vi "JSONtext Multi-step Filter.vi"() -> ()   [LabVIEW 2017] (continued)
53bcb93de39cd0c0af940\",\n    \"index\": 27,\n    \"guid\": \"0f0552d9-e7b3-4c57-b6c7-1e2135a1104f\",\n    \"isActive\": false,\n    \"balance\": \"$3,811.17\",\n    \"picture\": \"http://placehold.it/32x32\",\n    \"age\": 38,\n    \"eyeColor\": \"brown\",\n    \"name\": \"Merrill Ray\",\n    \"gender\": \"male\",\n    \"company\": \"SOLAREN\",\n    \"email\": \"merrillray@solaren.com\",\n    \"phone\": \"+1 (835) 524-2354\",\n    \"address\": \"227 Seacoast Terrace, Waterford, Kansas, 9740\",\n    \"about\": \"Magna eiusmod duis pariatur eiusmod minim et officia sit amet ipsum ut sint magna Lorem. Nisi velit sit adipisicing deserunt voluptate consectetur dolor officia voluptate elit adipisicing sit. Sint dolore occaecat ea duis voluptate duis sint ullamco in quis pariatur irure. Ipsum magna voluptate nulla deserunt eiusmod consectetur ut tempor qui pariatur quis duis. Lorem dolore qui adipisicing pariatur mollit cillum sunt nisi id deserunt tempor nisi amet. Sit cillum nisi dolore magna exercitation anim ad id consequat duis.\\r\\n\",\n    \"registered\": \"2016-06-15T02:30:18 -01:00\",\n    \"latitude\": 82.245484,\n    \"longitude\": -22.28782,\n    \"tags\": [\n      \"quis\",\n      \"pariatur\",\n      \"nisi\",\n      \"culpa\",\n      \"ut\",\n      \"minim\",\n      \"amet\"\n    ],\n    \"friends\": [\n      {\n        \"id\": 0,\n        \"name\": \"Fleming Rosario\"\n      },\n      {\n        \"id\": 1,\n        \"name\": \"Mcconnell Griffin\"\n      },\n      {\n        \"id\": 2,\n        \"name\": \"Marian Bradley\"\n      }\n    ],\n    \"greeting\": \"Hello, Merrill Ray! You have 3 unread messages.\",\n    \"favoriteFruit\": \"strawberry\"\n  },\n  {\n    \"_id\": \"59b53bcb56ebb2118edadabb\",\n    \"index\": 28,\n    \"guid\": \"31fd77e0-df37-4030-b598-6469f87deaaa\",\n    \"isActive\": false,\n    \"balance\": \"$1,128.38\",\n    \"picture\": \"http://placehold.it/32x32\",\n    \"age\": 22,\n    \"eyeColor\": \"green\",\n    \"name\": \"Cunningham Blevins\",\n    \"gender\": \"male\",\n    \"company\": \"SHOPABOUT\",\n    \"email\": \"cunninghamblevins@shopabout.com\",\n    \"phone\": \"+1 (960) 458-2822\",\n    \"address\": \"730 Llama Court, Riner, Puerto Rico, 7836\",\n    \"about\": \"Dolor quis officia nulla dolor amet sint excepteur enim esse est do. Eu ex ut aliquip velit do sint ullamco laborum. Occaecat eiusmod eiusmod velit adipisicing sit. Mollit eu pariatur eu consequat dolore irure fugiat sunt eiusmod cillum duis adipisicing eiusmod. Do commodo nisi irure cillum magna nulla enim aliqua dolor ullamco dolore pariatur.\\r\\n\",\n    \"registered\": \"2016-09-06T04:22:46 -01:00\",\n    \"latitude\": 83.759644,\n    \"longitude\": -43.131498,\n    \"tags\": [\n      \"velit\",\n      \"fugiat\",\n      \"dolor\",\n      \"ad\",\n      \"elit\",\n      \"dolore\",\n      \"ea\"\n    ],\n    \"friends\": [\n      {\n        \"id\": 0,\n        \"name\": \"Sanford Shannon\"\n      },\n      {\n        \"id\": 1,\n        \"name\": \"Burt Cherry\"\n      },\n      {\n        \"id\": 2,\n        \"name\": \"Kline Hale\"\n      }\n    ],\n    \"greeting\": \"Hello, Cunningham Blevins! You have 10 unread messages.\",\n    \"favoriteFruit\": \"strawberry\"\n  },\n  {\n    \"_id\": \"59b53bcb90a0cd7d08d9bf70\",\n    \"index\": 29,\n    \"guid\": \"8fb07447-f204-4b08-975d-44052bc193eb\",\n    \"isActive\": false,\n    \"balance\": \"$3,739.37\",\n    \"picture\": \"http://placehold.it/32x32\",\n    \"age\": 36,\n    \"eyeColor\": \"brown\",\n    \"name\": \"Bonner Lane\",\n    \"gender\": \"male\",\n    \"company\": \"COMVEY\",\n    \"email\": \"bonnerlane@comvey.com\",\n    \"phone\": \"+1 (847) 514-2794\",\n    \"address\": \"269 Dupont Street, Cedarville, South Carolina, 6587\",\n    \"about\": \"Velit Lorem magna deserunt minim ea exercitation quis veniam. Culpa cillum do aliquip exercitation enim aute in incididunt nostrud esse nostrud ullamco in. Amet mollit laborum eu laborum magna. Duis ad proident cillum esse fugiat enim est sit commodo. Dolore consectetur ut duis deserunt elit aliqua ad fugiat consectetur. Est aute aliquip ea consequat reprehenderit eiusmod. Consectetur tempor consequat duis voluptate mollit elit labore voluptate do cillum ex.\\r\\n\",\n    \"registered\": \"2017-02-20T02:31:32 -00:00\",\n    \"latitude\": -71.168208,\n    \"longitude\": -127.709761,\n    \"tags\": [\n      \"voluptate\",\n      \"consequat\",\n      \"incididunt\",\n      \"occaecat\",\n      \"amet\",\n      \"consequat\",\n      \"id\"\n    ],\n    \"friends\": [\n      {\n        \"id\": 0,\n        \"name\": \"Josie Horne\"\n      },\n      {\n        \"id\": 1,\n        \"name\": \"Nichole Weiss\"\n      },\n      {\n        \"id\": 2,\n        \"name\": \"Kristina Davidson\"\n      }\n    ],\n    \"greeting\": \"Hello, Bonner Lane! You have 3 unread messages.\",\n    \"favoriteFruit\": \"apple\"\n  },\n  {\n    \"_id\": \"59b53bcb35a25f2270b16071\",\n    \"index\": 30,\n    \"guid\": \"267938cb-8119-471f-85af-aa7a668d65fd\",\n    \"isActive\": false,\n    \"balance\": \"$2,354.36\",\n    \"picture\": \"http://placehold.it/32x32\",\n    \"age\": 35,\n    \"eyeColor\": \"blue\",\n    \"name\": \"Nielsen Burnett\",\n    \"gender\": \"male\",\n    \"company\": \"TURNABOUT\",\n    \"email\": \"nielsenburnett@turnabout.com\",\n    \"phone\": \"+1 (901) 404-2369\",\n    \"address\": \"499 Hart Place, Chesterfield, Mississippi, 6896\",\n    \"about\": \"Sunt magna sint ea deserunt reprehenderit aliqua in et proident. Minim consectetur dolore et commodo. Voluptate consectetur qui occaecat dolore eiusmod proident fugiat aute nulla id ad culpa exercitation occaecat.\\r\\n\",\n    \"registered\": \"2015-02-20T12:03:11 -00:00\",\n    \"latitude\": -46.775808,\n    \"longitude\": 173.193033,\n    \"tags\": [\n      \"enim\",\n      \"dolor\",\n      \"duis\",\n      \"Lorem\",\n      \"in\",\n      \"reprehenderit\",\n      \"ullamco\"\n    ],\n    \"friends\": [\n      {\n        \"id\": 0,\n        \"name\": \"Barlow Mcfadden\"\n      },\n      {\n        \"id\": 1,\n        \"name\": \"Clarissa Charles\"\n      },\n      {\n        \"id\": 2,\n        \"name\": \"Bray Patel\"\n      }\n    ],\n    \"greeting\": \"Hello, Nielsen Burnett! You have 7 unread messages.\",\n    \"favoriteFruit\": \"strawberry\"\n  },\n  {\n    \"_id\": \"59b53bcbe85d478fcadd3603\",\n    \"index\": 31,\n    \"guid\": \"3be04d8f-e807-4ad6-8ebd-c23cdbfe3dc4\",\n    \"isActive\": false,\n    \"balance\": \"$1,972.40\",\n    \"picture\": \"http://placehold.it/32x32\",\n    \"age\": 37,\n    \"eyeColor\": \"blue\",\n    \"name\": \"Elaine Allison\",\n    \"gender\": \"female\",\n    \"company\": \"QUANTASIS\",\n    \"email\": \"elaineallison@quantasis.com\",\n    \"phone\": \"+1 (981) 596-2824\",\n    \"address\": \"921 Kent Avenue, Breinigsville, Wisconsin, 3750\",\n    \"about\": \"Minim cillum ea irure officia. Irure in dolor ea veniam adipisicing sint nisi amet ipsum excepteur nisi excepteur est deserunt. Consequat voluptate mollit sint magna Lorem in nulla proident Lorem. Proident est id esse ad ea. Dolore Lorem aliquip officia veniam anim velit et id ullamco et dolor eu aliqua quis. Dolore magna est mollit in ut ea voluptate nostrud do aliquip. In reprehenderit non eiusmod veniam ex.\\r\\n\",\n    \"registered\": \"2017-03-24T04:15:39 -00:00\",\n    \"latitude\": 7.656665,\n    \"longitude\": 56.755826,\n    \"tags\": [\n      \"nisi\",\n      \"labore\",\n      \"fugiat\",\n      \"ex\",\n      \"reprehenderit\",\n      \"nisi\",\n      \"sint\"\n    ],\n    \"friends\": [\n      {\n        \"id\": 0,\n        \"name\": \"Alta Bruce\"\n      },\n      {\n        \"id\": 1,\n        \"name\": \"Cora Ruiz\"\n      },\n      {\n        \"id\": 2,\n        \"name\": \"Mercer Barron\"\n      }\n    ],\n    \"greeting\": \"Hello, Elaine Allison! You have 1 unread messages.\",\n    \"favoriteFruit\": \"banana\"\n  },\n  {\n    \"_id\": \"59b53bcbf5dcc9341b3c298d\",\n    \"index\": 32,\n    \"guid\": \"bf62375b-123f-4c02-85e3-3a78c18e6f70\",\n    \"isActive\": false,\n    \"balance\": \"$1,895.96\",\n    \"picture\": \"http://placehold.it/32x32\",\n    \"age\": 28,\n    \"eyeColor\": \"brown\",\n    \"name\": \"Christa Robertson\",\n    \"gender\": \"female\",\n    \"company\": \"ICOLOGY\",\n    \"email\": \"christarobertson@icology.com\",\n    \"phone\": \"+1 (888) 410-3337\",\n    \"address\": \"989 Clara Street, Ogema, Indiana, 2922\",\n    \"about\": \"Enim mollit officia occaecat non nostrud ad cupidatat amet. Sunt ipsum proident consectetur voluptate id excepteur id magna. Do commodo culpa id esse officia cupidatat dolore duis non laboris veniam. Laboris ad dolor qui anim et ut dolor excepteur irure elit adipisicing ex labore eiusmod. Sunt minim velit nostrud irure quis consequat officia fugiat amet ipsum. Nostrud laboris do fugiat proident reprehenderit duis exercitation aute enim ex ullamco proident. Qui sint adipisicing occaecat aliqua non culpa esse id dolor voluptate ipsum deserunt in.\\r\\n\",\n    \"registered\": \"2015-02-16T07:12:55 -00:00\",\n    \"latitude\": 52.102423,\n    \"longitude\": -24.794434,\n    \"tags\": [\n      \"dolore\",\n      \"fugiat\",\n      \"aliqua\",\n      \"minim\",\n      \"pariatur\",\n      \"laborum\",\n      \"qui\"\n    ],\n    \"friends\": [\n      {\n        \"id\": 0,\n        \"name\": \"Cathy Cohen\"\n      },\n      {\n        \"id\": 1,\n        \"name\": \"Shawna Green\"\n      },\n      {\n        \"id\": 2,\n        \"name\": \"Ward Mckay\"\n      }\n    ],\n    \"greeting\": \"Hello, Christa Robertson! You have 9 unread messages.\",\n    \"favoriteFruit\": \"banana\"\n  },\n  {\n    \"_id\": \"59b53bcb8f369a2e50811288\",\n    \"index\": 33,\n    \"guid\": \"74275f14-281e-4519-a0c4-b708fa901d88\",\n    \"isActive\": true,\n    \"balance\": \"$2,269.82\",\n    \"picture\": \"http://placehold.it/32x32\",\n    \"age\": 36,\n    \"eyeColor\": \"green\",\n    \"name\": \"Castillo Kerr\",\n    \"gender\": \"male\",\n    \"company\": \"ZENTHALL\",\n    \"email\": \"castillokerr@zenthall.com\",\n    \"phone\": \"+1 (964) 406-2670\",\n    \"address\": \"210 Campus Road, Templeton, Tennessee, 2482\",\n    \"about\": \"Irure ut nisi adipisicing non duis mollit. Tempor deserunt ut nostrud ipsum enim dolore Lorem labore. Duis sint magna nisi et anim ex. Ea eu exercitation est laboris nostrud qui eiusmod. Ullamco amet ut Lorem eu adipisicing incididunt qui aliquip pariatur sint proident anim voluptate veniam. Excepteur aute velit deserunt deserunt et ex elit excepteur enim reprehenderit. Commodo ad aliquip Lorem excepteur reprehenderit quis in ea sint esse proident.\\r\\n\",\n    \"registered\": \"2016-05-03T04:24:26 -01:00\",\n    \"latitude\": -38.877683,\n    \"longitude\": -171.766918,\n    \"tags\": [\n      \"officia\",\n      \"aliquip\",\n      \"consequat\",\n      \"voluptate\",\n      \"cillum\",\n      \"do\",\n      \"officia\"\n    ],\n    \"friends\": [\n      {\n        \"id\": 0,\n        \"name\": \"Cara Hoffman\"\n      },\n      {\n        \"id\": 1,\n        \"name\": \"Joyner Beasley\"\n      },\n      {\n        \"id\": 2,\n        \"name\": \"Lucy Grimes\"\n      }\n    ],\n    \"greeting\": \"Hello, Castillo Kerr! You have 9 unread messages.\",\n    \"favoriteFruit\": \"strawberry\"\n  },\n  {\n    \"_id\": \"59b53bcbb2ac6162cf8d89a7\",\n    \"index\": 34,\n    \"guid\": \"3d62cd17-ac67-4b71-a5da-4ccef6cce1d0\",\n    \"isActive\": false,\n    \"balance\": \"$1,731.00\",\n    \"picture\": \"http://placehold.it/32x32\",\n    \"age\": 24,\n    \"eyeColor\": \"blue\",\n    \"name\": \"Melissa Gregory\",\n    \"gender\": \"female\",\n    \"company\": \"UPLINX\",\n    \"email\": \"melissagregory@uplinx.com\",\n    \"phone\": \"+1 (907) 532-2994\",\n    \"address\": \"394 Miller Avenue, Cashtown, Georgia, 520\",\n    \"about\": \"Consequat mollit occaecat proident officia reprehenderit. Ipsum minim ex reprehenderit et reprehenderit sunt. Esse ea quis nulla do. Cupidatat sit et tempor tempor voluptate qui est ad. Ad magna adipisicing excepteur excepteur ad quis. Fugiat laborum adipisicing do commodo ex qui ut minim ipsum commodo irure ex ea. Fugiat ad anim dolor do adipisicing veniam laboris laboris nostrud reprehenderit mollit eiusmod dolore laboris.\\r\\n\",\n    \"registered\": \"2016-03-22T12:23:21 -00:00\",\n    \"latitude\": -13.24058,\n    \"longitude\": 174.343852,\n    \"tags\": [\n      \"aliqua\",\n      \"veniam\",\n      \"do\",\n      \"tempor\",\n      \"voluptate\",\n      \"officia\",\n      \"id\"\n    ],\n    \"friends\": [\n      {\n        \"id\": 0,\n        \"name\": \"Mccall Baker\"\n      },\n      {\n        \"id\": 1,\n        \"name\": \"Elena Raymond\"\n      },\n      {\n        \"id\": 2,\n        \"name\": \"Harvey Hubbard\"\n      }\n    ],\n    \"greeting\": \"Hello, Melissa Gregory! You have 7 unread messages.\",\n    \"favoriteFruit\": \"banana\"\n  },\n  {\n    \"_id\": \"59b53bcb9bea1476ae4824c8\",\n    \"index\": 35,\n    \"guid\": \"705c7090-a759-43dc-b18c-63ad736d29ca\",\n    \"isActive\": false,\n    \"balance\": \"$2,004.78\",\n    \"picture\": \"http://placehold.it/32x32\",\n    \"age\": 37,\n    \"eyeColor\": \"brown\",\n    \"name\": \"Lancaster Welch\",\n    \"gender\": \"male\",\n    \"company\": \"JIMBIES\",\n    \"email\": \"lancasterwelch@jimbies.com\",\n    \"phone\": \"+1 (961) 509-2893\",\n    \"address\": \"477 Crystal Street, Lindcove, New Hampshire, 655\",\n    \"about\": \"Anim ex duis laboris non ullamco non deserunt magna ex voluptate mollit in excepteur. Sit excepteur proident ad magna esse elit veniam qui ad veniam cupidatat non duis. Eiusmod laboris id cupidatat exercitation quis adipisicing sunt eiusmod enim magna. Qui aliqua qui dolore enim veniam consequat ea cillum cupidatat voluptate excepteur in. Eu culpa anim veniam nisi officia consectetur ut exercitation fugiat quis sit ipsum enim quis. Lorem ut magna in sit.\\r\\n\",\n    \"registered\": \"2016-07-01T05:06:00 -01:00\",\n    \"latitude\": 29.49636,\n    \"longitude\": -45.617538,\n    \"tags\": [\n      \"adipisicing\",\n      \"enim\",\n      \"do\",\n      \"culpa\",\n      \"esse\",\n      \"proident\",\n      \"velit\"\n    ],\n    \"friends\": [\n      {\n        \"id\": 0,\n        \"name\": \"Whitehead Moss\"\n      },\n      {\n        \"id\": 1,\n        \"name\": \"Melisa Bridges\"\n      },\n      {\n        \"id\": 2,\n        \"name\": \"Helene Barrett\"\n      }\n    ],\n    \"greeting\": \"Hello, Lancaster Welch! You have 4 unread messages.\",\n    \"favoriteFruit\": \"strawberry\"\n  },\n  {\n    \"_id\": \"59b53bcb1dfb6733db2fc827\",\n    \"index\": 36,\n    \"guid\": \"0d80f8b7-650a-4492-b9ae-8c5d36bf2d83\",\n    \"isActive\": true,\n    \"balance\": \"$3,087.53\",\n    \"picture\": \"http://placehold.it/32x32\",\n    \"age\": 21,\n    \"eyeColor\": \"brown\",\n    \"name\": \"Clemons Juarez\",\n    \"gender\": \"male\",\n    \"company\": \"EMERGENT\",\n    \"email\": \"clemonsjuarez@emergent.com\",\n    \"phone\": \"+1 (899) 574-2444\",\n    \"address\": \"962 Seagate Avenue, Diaperville, Louisiana, 9282\",\n    \"about\": \"Labore adipisicing in enim eu laboris veniam minim sit do velit. Nulla amet ullamco anim cupidatat. Aliquip officia laborum nulla nisi aliqua dolore elit aute tempor ut culpa commodo. Esse cupidatat officia pariatur pariatur.\\r\\n\",\n    \"registered\": \"2015-07-29T04:09:12 -01:00\",\n    \"latitude\": 16.025236,\n    \"longitude\": -68.678922,\n    \"tags\": [\n      \"et\",\n      \"sunt\",\n      \"enim\",\n      \"dolor\",\n      \"labore\",\n      \"nostrud\",\n      \"adipisicing\"\n    ],\n    \"friends\": [\n      {\n        \"id\": 0,\n        \"name\": \"Dorothea Barnett\"\n      },\n      {\n        \"id\": 1,\n        \"name\": \"Terrie Knox\"\n      },\n      {\n        \"id\": 2,\n        \"name\": \"Dodson Dale\"\n      }\n    ],\n    \"greeting\": \"Hello, Clemons Juarez! You have 7 unread messages.\",\n    \"favoriteFruit\": \"apple\"\n  },\n  {\n    \"_id\": \"59b53bcba7232f419ad64f14\",\n    \"index\": 37,\n    \"guid\": \"15bec63f-2a77-45db-a3cf-11092f20cb9e\",\n    \"isActive\": false,\n    \"balance\": \"$3,716.74\",\n    \"picture\": \"http://placehold.it/32x32\",\n    \"age\": 29,\n    \"eyeColor\": \"green\",\n    \"name\": \"Hillary Waller\",\n    \"gender\": \"female\",\n    \"company\": \"MUSIX\",\n    \"email\": \"hillarywaller@musix.com\",\n    \"phone\": \"+1 (947) 549-3976\",\n    \"address\": \"601 Kay Court, Rockhill, Oklahoma, 5198\",\n    \"about\": \"Sit reprehenderit ad mollit reprehenderit do aliquip fugiat aute consectetur eu excepteur eiusmod dolor Lorem. Deserunt consectetur ex et deserunt velit quis excepteur labore deserunt cillum. Dolore mollit qui proident minim eiusmod.\\r\\n\",\n    \"registered\": \"2015-10-22T03:23:57 -01:00\",\n    \"latitude\": 2.128634,\n    \"longitude\": 43.198503,\n    \"tags\": [\n      \"duis\",\n      \"non\",\n      \"dolore\",\n      \"aliqua\",\n      \"culpa\",\n      \"proident\",\n      \"sint\"\n    ],\n    \"friends\": [\n      {\n        \"id\": 0,\n        \"name\": \"Vega Lawson\"\n      },\n      {\n        \"id\": 1,\n        \"name\": \"Phelps Wolf\"\n      },\n      {\n        \"id\": 2,\n        \"name\": \"Gloria Mcmillan\"\n      }\n    ],\n    \"greeting\": \"Hello, Hillary Waller! You have 10 unread messages.\",\n    \"favoriteFruit\": \"apple\"\n  },\n  {\n    \"_id\": \"59b53bcb1344ea6331b52625\",\n    \"index\": 38,\n    \"guid\": \"561edd27-6d57-4a6f-956c-f3bf54efe435\",\n    \"isActive\": true,\n    \"balance\": \"$3,213.23\",\n    \"picture\": \"http://placehold.it/32x32\",\n    \"age\": 32,\n    \"eyeColor\": \"brown\",\n    \"name\": \"Jackie Lott\",\n    \"gender\": \"female\",\n    \"company\": \"ORBIN\",\n    \"email\": \"jackielott@orbin.com\",\n    \"phone\": \"+1 (825) 509-2344\",\n    \"address\": \"921 Frost Street, Dubois, Alaska, 1796\",\n    \"about\": \"Reprehenderit veniam Lorem ea do proident in fugiat aliqua. Id proident nostrud aliqua tempor reprehenderit eiusmod ullamco velit duis. Anim ipsum nulla reprehenderit do exercitation consequat nisi in commodo qui fugiat nostrud.\\r\\n\",\n    \"registered\": \"2017-08-19T04:32:54 -01:00\",\n    \"latitude\": 23.292166,\n    \"longitude\": 35.845555,\n    \"tags\": [\n      \"dolore\",\n      \"veniam\",\n      \"labore\",\n      \"et\",\n      \"culpa\",\n      \"est\",\n      \"officia\"\n    ],\n    \"friends\": [\n      {\n        \"id\": 0,\n        \"name\": \"Diaz Warren\"\n      },\n      {\n        \"id\": 1,\n        \"name\": \"Sullivan Watkins\"\n      },\n      {\n        \"id\": 2,\n        \"name\": \"Maynard Page\"\n      }\n    ],\n    \"greeting\": \"Hello, Jackie Lott! You have 4 unread messages.\",\n    \"favoriteFruit\": \"apple\"\n  },\n  {\n    \"_id\": \"59b53bcb21e1aba2d54ad2f8\",\n    \"index\": 39,\n    \"guid\": \"c9ee8206-d3bd-48ae-9fda-5b5529ac4057\",\n    \"isActive\": false,\n    \"balance\": \"$3,035.61\",\n    \"picture\": \"http://placehold.it/32x32\",\n    \"age\": 29,\n    \"eyeColor\": \"green\",\n    \"name\": \"Flynn Pruitt\",\n    \"gender\": \"male\",\n    \"company\": \"ORBEAN\",\n    \"email\": \"flynnpruitt@orbean.com\",\n    \"phone\": \"+1 (866) 596-2533\",\n    \"address\": \"274 Ridgewood Place, Durham, North Dakota, 3534\",\n    \"about\": \"Commodo sint irure deserunt Lorem laboris laborum mollit ea ipsum incididunt laboris adipisicing proident. Velit tempor minim et occaecat exercitation et commodo consequat velit. Minim irure esse ullamco commodo labore ex mollit esse. Ipsum nostrud est ex Lorem culpa.\\r\\n\",\n    \"registered\": \"2015-06-20T09:17:37 -01:00\",\n    \"latitude\": -50.018521,\n    \"longitude\": 165.121492,\n    \"tags\": [\n      \"irure\",\n      \"ea\",\n      \"quis\",\n      \"dolore\",\n      \"irure\",\n      \"aliqua\",\n      \"pariatur\"\n    ],\n    \"friends\": [\n      {\n        \"id\": 0,\n        \"name\": \"Carla Snow\"\n      },\n      {\n        \"id\": 1,\n        \"name\": \"Cochran Thomas\"\n      },\n      {\n        \"id\": 2,\n        \"name\": \"Guy Roberts\"\n      }\n    ],\n    \"greeting\": \"Hello, Flynn Pruitt! You have 10 unread messages.\",\n    \"favoriteFruit\": \"banana\"\n  },\n  {\n    \"_id\": \"59b53bcb88a5fd7e5b5805c7\",\n    \"index\": 40,\n    \"guid\": \"ef10c0b3-7ab0-4313-b2b2-462164f5485a\",\n    \"isActive\": true,\n    \"balance\": \"$1,173.28\",\n    \"picture\": \"http://placehold.it/32x32\",\n    \"age\": 39,\n    \"eyeColor\": \"brown\",\n    \"name\": \"Shelby Albert\",\n    \"gender\": \"female\",\n    \"company\": \"HYDROCOM\",\n    \"email\": \"shelbyalbert@hydrocom.com\",\n    \"phone\": \"+1 (977) 400-2351\",\n    \"address\": \"393 Glendale Court, Catharine, Washington, 6629\",\n    \"about\": \"Do laborum exercitation eiusmod sunt esse laboris qui Lorem dolor amet consectetur id. Officia est exercitation proident pariatur culpa ea sint veniam reprehenderit aliquip. Laborum dolore ad mollit nostrud cillum ad tempor anim occaecat sit. Amet consequat eiusmod laboris consectetur.\\r\\n\",\n    \"registered\": \"2015-07-17T06:49:02 -01:00\",\n    \"latitude\": -32.156776,\n    \"longitude\": -68.42255,\n    \"tags\": [\n      \"laborum\",\n      \"dolor\",\n      \"sit\",\n      \"sit\",\n      \"ad\",\n      \"sunt\",\n      \"minim\"\n    ],\n    \"friends\": [\n      {\n        \"id\": 0,\n        \"name\": \"Huber Hahn\"\n      },\n      {\n        \"id\": 1,\n        \"name\": \"Felicia Mooney\"\n      },\n      {\n        \"id\": 2,\n        \"name\": \"Kathryn Alvarado\"\n      }\n    ],\n    \"greeting\": \"Hello, Shelby Albert! You have 1 unread messages.\",\n    \"favoriteFruit\": \"banana\"\n  },\n  {\n    \"_id\": \"59b53bcbacd63a0258d513a3\",\n    \"index\": 41,\n    \"guid\": \"7142ec6a-9741-41fd-8c8f-fba9cc5ff0ab\",\n    \"isActive\": true,\n    \"balance\": \"$3,196.96\",\n    \"picture\": \"http://placehold.it/32x32\",\n    \"age\": 34,\n    \"eyeColor\": \"brown\",\n    \"name\": \"Bailey Snyder\",\n    \"gender\": \"male\",\n    \"company\": \"ISOSURE\",\n    \"email\": \"baileysnyder@isosure.com\",\n    \"phone\": \"+1 (976) 469-3334\",\n    \"address\": \"754 Emerson Place, Stagecoach, New York, 1029\",\n    \"about\": \"Veniam dolore qui elit ea qui ipsum exercitation sunt sunt in ad mollit. Excepteur adipisicing et consectetur proident veniam laborum adipisicing consectetur eiusmod. Culpa consequat officia ipsum nisi proident proident velit. Fugiat commodo ad do commodo tempor proident excepteur mollit magna.\\r\\n\",\n    \"registered\": \"2015-09-25T01:25:56 -01:00\",\n    \"latitude\": -76.0324,\n    \"longitude\": -73.748444,\n    \"tags\": [\n      \"minim\",\n      \"adipisicing\",\n      \"Lorem\",\n      \"eu\",\n      \"ex\",\n      \"deserunt\",\n      \"eu\"\n    ],\n    \"friends\": [\n      {\n        \"id\": 0,\n        \"name\": \"Waters Hartman\"\n      },\n      {\n        \"id\": 1,\n        \"name\": \"Valdez Baird\"\n      },\n      {\n        \"id\": 2,\n        \"name\": \"Serena Mills\"\n      }\n    ],\n    \"greeting\": \"Hello, Bailey Snyder! You have 5 unread messages.\",\n    \"favoriteFruit\": \"strawberry\"\n  },\n  {\n    \"_id\": \"59b53bcba4a6b906f6c552ad\",\n    \"index\": 42,\n    \"guid\": \"46d7ec6e-a1f2-4133-bd5d-cc56e5102a00\",\n    \"isActive\": true,\n    \"balance\": \"$3,341.48\",\n    \"picture\": \"http://placehold.it/32x32\",\n    \"age\": 32,\n    \"eyeColor\": \"brown\",\n    \"name\": \"Erika Porter\",\n    \"gender\": \"female\",\n    \"company\": \"ZENTIME\",\n    \"email\": \"erikaporter@zentime.com\",\n    \"phone\": \"+1 (937) 468-3114\",\n    \"address\": \"917 Ovington Avenue, Stouchsburg, Alabama, 9680\",\n    \"about\": \"Consectetur reprehenderit nisi cupidatat deserunt nulla laboris ut. Nisi deserunt dolore occaecat fugiat esse pariatur quis non commodo laboris elit voluptate. Nulla ex laborum Lorem ipsum incididunt reprehenderit elit dolore ullamco amet duis esse est ullamco. Enim in mollit labore laborum sunt.\\r\\n\",\n    \"registered\": \"2015-01-22T11:40:33 -00:00\",\n    \"latitude\": 53.845955,\n    \"longitude\": -126.430992,\n    \"tags\": [\n      \"incididunt\",\n      \"elit\",\n      \"duis\",\n      \"deserunt\",\n      \"sint\",\n      \"labore\",\n      \"irure\"\n    ],\n    \"friends\": [\n      {\n        \"id\": 0,\n        \"name\": \"Monica Lyons\"\n      },\n      {\n        \"id\": 1,\n        \"name\": \"Katrina Brennan\"\n      },\n      {\n        \"id\": 2,\n        \"name\": \"Kim Francis\"\n      }\n    ],\n    \"greeting\": \"Hello, Erika Porter! You have 4 unread messages.\",\n    \"favoriteFruit\": \"strawberry\"\n  },\n  {\n    \"_id\": \"59b53bcb1c73edcfc9efe849\",\n    \"index\": 43,\n    \"guid\": \"84a42cb7-4fea-42c7-961d-2535547c818b\",\n    \"isActive\": true,\n    \"balance\": \"$1,840.08\",\n    \"picture\": \"http://placehold.it/32x32\",\n    \"age\": 29,\n    \"eyeColor\": \"brown\",\n    \"name\": \"Marjorie Craig\",\n    \"gender\": \"female\",\n    \"company\": \"PROGENEX\",\n    \"email\": \"marjoriecraig@progenex.com\",\n    \"phone\": \"+1 (898) 534-3929\",\n    \"address\": \"262 Exeter Street, Elliott, Arkansas, 9839\",\n    \"about\": \"Ipsum esse irure dolor consectetur amet ullamco. Ut nostrud anim occaecat dolor dolor sit adipisicing cupidatat. Veniam velit pariatur id magna in sit.\\r\\n\",\n    \"registered\": \"2014-11-10T05:13:50 -00:00\",\n    \"latitude\": 74.482858,\n    \"longitude\": 69.078973,\n    \"tags\": [\n      \"excepteur\",\n      \"cillum\",\n      \"minim\",\n      \"aliqua\",\n      \"exercitation\",\n      \"incididunt\",\n      \"dolor\"\n    ],\n    \"friends\": [\n      {\n        \"id\": 0,\n        \"name\": \"Horton Taylor\"\n      },\n      {\n        \"id\": 1,\n        \"name\": \"Melinda Ashley\"\n      },\n      {\n        \"id\": 2,\n        \"name\": \"Margie Roy\"\n      }\n    ],\n    \"greeting\": \"Hello, Marjorie Craig! You have 6 unread messages.\",\n    \"favoriteFruit\": \"banana\"\n  },\n  {\n    \"_id\": \"59b53bcb2edcfd9a5f058115\",\n    \"index\": 44,\n    \"guid\": \"8101a8ef-a578-4a86-9b90-204b2b6ca3bc\",\n    \"isActive\": false,\n    \"balance\": \"$1,295.45\",\n    \"picture\": \"http://placehold.it/32x32\",\n    \"age\": 20,\n    \"eyeColor\": \"blue\",\n    \"name\": \"Tina Browning\",\n    \"gender\": \"female\",\n    \"company\": \"KNOWLYSIS\",\n    \"email\": \"tinabrowning@knowlysis.com\",\n    \"phone\": \"+1 (878) 557-2240\",\n    \"address\": \"470 Lawton Street, Avoca, Northern Mariana Islands, 1174\",\n    \"about\": \"Officia quis reprehenderit eiusmod sit mollit duis minim duis elit exercitation sunt quis aliquip est. Velit esse occaecat irure deserunt amet dolore voluptate deserunt exercitation id. Dolor culpa dolor adipisicing do irure. Ullamco incididunt elit non mollit excepteur nisi proident ut eu sit dolor excepteur. Reprehenderit Lorem adipisicing deserunt eu labore laborum cillum ullamco nisi esse magna. Amet et ad nisi ad elit velit in in sunt veniam occaecat pariatur quis exercitation.\\r\\n\",\n    \"registered\": \"2015-10-18T08:14:25 -01:00\",\n    \"latitude\": 35.369634,\n    \"longitude\": -88.568524,\n    \"tags\": [\n      \"eu\",\n      \"veniam\",\n      \"quis\",\n      \"sint\",\n      \"excepteur\",\n      \"fugiat\",\n      \"minim\"\n    ],\n    \"friends\": [\n      {\n        \"id\": 0,\n        \"name\": \"Yolanda Mcgee\"\n      },\n      {\n        \"id\": 1,\n        \"name\": \"Tara Rich\"\n      },\n      {\n        \"id\": 2,\n        \"name\": \"Walton Maynard\"\n      }\n    ],\n    \"greeting\": \"Hello, Tina Browning! You have 8 unread messages.\",\n    \"favoriteFruit\": \"apple\"\n  },\n  {\n    \"_id\": \"59b53bcb3e923247d8ec4740\",\n    \"index\": 45,\n    \"guid\": \"b966f77e-3e7a-4bc1-8268-d15e38d760e2\",\n    \"isActive\": false,\n    \"balance\": \"$1,071.05\",\n    \"picture\": \"http://placehold.it/32x32\",\n    \"age\": 34,\n    \"eyeColor\": \"blue\",\n    \"name\": \"Estela Morrison\",\n    \"gender\": \"female\",\n    \"company\": \"DELPHIDE\",\n    \"email\": \"estelamorrison@delphide.com\",\n    \"phone\": \"+1 (895) 541-2685\",\n    \"address\": \"492 Ryder Avenue, Sims, West Virginia, 7864\",\n    \"about\": \"Est aliqua sit consectetur do occaecat ullamco commodo fugiat et. Culpa amet ipsum enim quis duis exercitation non nisi adipisicing aliquip incididunt irure. Labore aliqua sint nulla reprehenderit in reprehenderit tempor ullamco quis ipsum. Fugiat irure ut sit adipisicing cillum magna ad sit enim elit irure. Proident aliqua eu et anim est reprehenderit fugiat non. Commodo enim id nulla sit nisi. Excepteur tempor officia ipsum in pariatur.\\r\\n\",\n    \"registered\": \"2015-01-29T12:06:00 -00:00\",\n    \"latitude\": -31.693065,\n    \"longitude\": -53.009874,\n    \"tags\": [\n      \"magna\",\n      \"consequat\",\n      \"enim\",\n      \"velit\",\n      \"anim\",\n      \"velit\",\n      \"ad\"\n    ],\n    \"friends\": [\n      {\n        \"id\": 0,\n        \"name\": \"Callahan King\"\n      },\n      {\n        \"id\": 1,\n        \"name\": \"Key Wallace\"\n      },\n      {\n        \"id\": 2,\n        \"name\": \"Carney Arnold\"\n      }\n    ],\n    \"greeting\": \"Hello, Estela Morrison! You have 3 unread messages.\",\n    \"favoriteFruit\": \"apple\"\n  },\n  {\n    \"_id\": \"59b53bcb1526a6fceba75760\",\n    \"index\": 46,\n    \"guid\": \"5ef8b250-99fd-4d8e-99c0-bb5f3d3bdac3\",\n    \"isActive\": false,\n    \"balance\": \"$2,675.97\",\n    \"picture\": \"http://placehold.it/32x32\",\n    \"age\": 31,\n    \"eyeColor\": \"green\",\n    \"name\": \"Adela Ryan\",\n    \"gender\": \"female\",\n    \"company\": \"FLUMBO\",\n    \"email\": \"adelaryan@flumbo.com\",\n    \"phone\": \"+1 (906) 429-3206\",\n    \"address\": \"952 Richmond Street, Rodanthe, South Dakota, 2236\",\n    \"about\": \"Ea non aliquip fugiat Lorem magna pariatur excepteur officia qui quis officia occaecat quis est. Amet incididunt nisi duis commodo sint cillum tempor. Minim reprehenderit ut Lorem labore eu magna proident voluptate occaecat amet quis. Ipsum nulla ullamco ad enim duis velit eiusmod consectetur aliqua ad. Nisi aliquip esse proident nostrud officia non sit laboris amet excepteur dolor commodo ad. Cillum velit et ad aliquip esse mollit in enim tempor dolor. Aliqua esse excepteur mollit mollit.\\r\\n\",\n    \"registered\": \"2014-08-15T04:54:20 -01:00\",\n    \"latitude\": 49.702844,\n    \"longitude\": 154.358542,\n    \"tags\": [\n      \"nostrud\",\n      \"non\",\n      \"laboris\",\n      \"nostrud\",\n      \"eu\",\n      \"adipisicing\",\n      \"ad\"\n    ],\n    \"friends\": [\n      {\n        \"id\": 0,\n        \"name\": \"Moss Bright\"\n      },\n      {\n        \"id\": 1,\n        \"name\": \"Houston Glass\"\n      },\n      {\n        \"id\": 2,\n        \"name\": \"Cherry Moon\"\n      }\n    ],\n    \"greeting\": \"Hello, Adela Ryan! You have 2 unread messages.\",\n    \"favoriteFruit\": \"apple\"\n  },\n  {\n    \"_id\": \"59b53bcbb6aeae8f27f300a9\",\n    \"index\": 47,\n    \"guid\": \"8e8ffd1c-34dd-4984-9245-b4713cc73b00\",\n    \"isActive\": true,\n    \"balance\": \"$3,353.90\",\n    \"picture\": \"http://placehold.it/32x32\",\n    \"age\": 36,\n    \"eyeColor\": \"blue\",\n    \"name\": \"Cote Barlow\",\n    \"gender\": \"male\",\n    \"company\": \"BEZAL\",\n    \"email\": \"cotebarlow@bezal.com\",\n    \"phone\": \"+1 (987) 473-2295\",\n    \"address\": \"560 Emmons Avenue, Wolcott, Delaware, 8148\",\n    \"about\": \"Qui aliqua sit laboris eu consectetur commodo qui ullamco cupidatat id enim ex sit. Anim reprehenderit tempor ut fugiat. Sunt et consequat proident proident. Irure sunt adipisicing commodo do enim exercitation fugiat aliqua consequat anim do et sint. Enim excepteur reprehenderit deserunt pariatur do voluptate ullamco aliqua magna labore deserunt tempor id. Enim dolor nostrud qui ullamco cillum officia mollit.\\r\\n\",\n    \"registered\": \"2014-04-10T08:27:55 -01:00\",\n    \"latitude\": 66.218671,\n    \"longitude\": 64.565323,\n    \"tags\": [\n      \"magna\",\n      \"reprehenderit\",\n      \"velit\",\n      \"nulla\",\n      \"aliqua\",\n      \"quis\",\n      \"nisi\"\n    ],\n    \"friends\": [\n      {\n        \"id\": 0,\n        \"name\": \"Stark Yates\"\n      },\n      {\n        \"id\": 1,\n        \"name\": \"Ginger Wilkinson\"\n      },\n      {\n        \"id\": 2,\n        \"name\": \"Bradford Durham\"\n      }\n    ],\n    \"greeting\": \"Hello, Cote Barlow! You have 10 unread messages.\",\n    \"favoriteFruit\": \"apple\"\n  },\n  {\n    \"_id\": \"59b53bcbb025a60e792d23e8\",\n    \"index\": 48,\n    \"guid\": \"399c42d0-8971-45d8-ac59-af2f1ffaebd0\",\n    \"isActive\": true,\n    \"balance\": \"$3,820.26\",\n    \"picture\": \"http://placehold.it/32x32\",\n    \"age\": 32,\n    \"eyeColor\": \"brown\",\n    \"name\": \"Higgins Randall\",\n    \"gender\": \"male\",\n    \"company\": \"ECSTASIA\",\n    \"email\": \"higginsrandall@ecstasia.com\",\n    \"phone\": \"+1 (895) 474-3692\",\n    \"address\": \"325 John Street, Welch, Nebraska, 2056\",\n    \"about\": \"Cupidatat non minim occaecat proident enim consectetur occaecat Lorem duis ut. Quis incididunt nostrud amet ut laborum consequat aliquip excepteur. Dolor ipsum aute consectetur id quis Lorem culpa nostrud sint ipsum esse reprehenderit aliqua. Dolor id ex consequat nisi quis esse officia veniam. Sit amet cillum ea irure consectetur exercitation laboris culpa deserunt magna aute dolor. Cillum deserunt irure velit quis ipsum esse cillum cillum ullamco id.\\r\\n\",\n    \"registered\": \"2014-04-12T05:46:39 -01:00\",\n    \"latitude\": -75.882125,\n    \"longitude\": -169.69303,\n    \"tags\": [\n      \"deserunt\",\n      \"nostrud\",\n      \"do\",\n      \"est\",\n      \"laboris\",\n      \"excepteur\",\n      \"fugiat\"\n    ],\n    \"friends\": [\n      {\n        \"id\": 0,\n        \"name\": \"Tran Baldwin\"\n      },\n      {\n        \"id\": 1,\n        \"name\": \"James Joyner\"\n      },\n      {\n        \"id\": 2,\n        \"name\": \"Lessie Velez\"\n      }\n    ],\n    \"greeting\": \"Hello, Higgins Randall! You have 5 unread messages.\",\n    \"favoriteFruit\": \"banana\"\n  },\n  {\n    \"_id\": \"59b53bcb5f007cb90b5b92ad\",\n    \"index\": 49,\n    \"guid\": \"9ae4ab4d-ba1b-405e-a321-ccd78ef7b7e2\",\n    \"isActive\": true,\n    \"balance\": \"$3,496.51\",\n    \"picture\": \"http://placehold.it/32x32\",\n    \"age\": 39,\n    \"eyeColor\": \"blue\",\n    \"name\": \"Roach Mosley\",\n    \"gender\": \"male\",\n    \"company\": \"GADTRON\",\n    \"email\": \"roachmosley@gadtron.com\",\n    \"phone\": \"+1 (866) 580-2668\",\n    \"address\": \"709 Hendrickson Place, Mooresburg, California, 2507\",\n    \"about\": \"Et nostrud voluptate sunt laborum id enim irure pariatur ea anim ex Lorem est sint. Cupidatat aliqua fugiat proident sunt ea et non sint sint. Ut cupidatat aliquip magna ullamco sit ipsum duis mollit Lorem exercitation ut qui consectetur.\\r\\n\",\n    \"registered\": \"2016-08-14T07:34:15 -01:00\",\n    \"latitude\": 35.818251,\n    \"longitude\": -110.714479,\n    \"tags\": [\n      \"et\",\n      \"enim\",\n      \"fugiat\",\n      \"dolore\",\n      \"enim\",\n      \"voluptate\",\n      \"sit\"\n    ],\n    \"friends\": [\n      {\n        \"id\": 0,\n        \"name\": \"Olga Bryant\"\n      },\n      {\n        \"id\": 1,\n        \"name\": \"Patricia Gill\"\n      },\n      {\n        \"id\": 2,\n        \"name\": \"Mandy Gallagher\"\n      }\n    ],\n    \"greeting\": \"Hello, Roach Mosley! You have 2 unread messages.\",\n    \"favoriteFruit\": \"apple\"\n  },\n  {\n    \"_id\": \"59b53bcbc26b07d63737890c\",\n    \"index\": 50,\n    \"guid\": \"5b403f4d-e53f-470c-9842-b661322b636e\",\n    \"isActive\": false,\n    \"balance\": \"$2,414.71\",\n    \"picture\": \"http://placehold.it/32x32\",\n    \"age\": 22,\n    \"eyeColor\": \"green\",\n    \"name\": \"Cleo Glenn\",\n    \"gender\": \"female\",\n    \"company\": \"OVERPLEX\",\n    \"email\": \"cleoglenn@overplex.com\",\n    \"phone\": \"+1 (814) 562-3233\",\n    \"address\": \"181 Grand Street, Bawcomville, Ohio, 9691\",\n    \"about\": \"Laboris dolor ullamco ad elit mollit magna. Ipsum velit cillum et sint ut ipsum voluptate ea commodo cupidatat pariatur ipsum irure. Ad nostrud sit Lorem ex proident irure.\\r\\n\",\n    \"registered\": \"2016-02-16T07:07:22 -00:00\",\n    \"latitude\": -8.199302,\n    \"longitude\": 101.098002,\n    \"tags\": [\n      \"consequat\",\n      \"voluptate\",\n      \"enim\",\n      \"sint\",\n      \"Lorem\",\n      \"cupidatat\",\n      \"ipsum\"\n    ],\n    \"friends\": [\n      {\n        \"id\": 0,\n        \"name\": \"Ollie Stafford\"\n      },\n      {\n        \"id\": 1,\n        \"name\": \"Meredith Terrell\"\n      },\n      {\n        \"id\": 2,\n        \"name\": \"Mcgee Salazar\"\n      }\n    ],\n    \"greeting\": \"Hello, Cleo Glenn! You have 9 unread messages.\",\n    \"favoriteFruit\": \"banana\"\n  },\n  {\n    \"_id\": \"59b53bcb235cd8621ba76b75\",\n    \"index\": 51,\n    \"guid\": \"d05378a5-ec58-4631-9007-10eb3f9b63c4\",\n    \"isActive\": true,\n    \"balance\": \"$2,009.31\",\n    \"picture\": \"http://placehold.it/32x32\",\n    \"age\": 38,\n    \"eyeColor\": \"blue\",\n    \"name\": \"Little Beck\",\n    \"gender\": \"male\",\n    \"company\": \"GOGOL\",\n    \"email\": \"littlebeck@gogol.com\",\n    \"phone\": \"+1 (928) 571-3851\",\n    \"address\": \"709 Willmohr Street, Jenkinsville, Federated States Of Micronesia, 8660\",\n    \"about\": \"Exercitation occaecat minim aute ex quis in qui ex cillum aute velit. Velit qui sunt velit exercitation veniam incididunt culpa nostrud do tempor non eiusmod. Ad do ad velit eiusmod laborum laboris reprehenderit occaecat tempor do. Excepteur laboris consectetur id occaecat qui cupidatat enim ullamco anim anim. Laborum occaecat dolor aliqua ipsum dolor labore in elit sit.\\r\\n\",\n    \"registered\": \"2014-06-22T01:39:32 -01:00\",\n    \"latitude\": 38.221291,\n    \"longitude\": -172.966121,\n    \"tags\": [\n      \"labore\",\n      \"ullamco\",\n      \"mollit\",\n      \"pariatur\",\n      \"quis\",\n      \"ipsum\",\n      \"qui\"\n    ],\n    \"friends\": [\n      {\n        \"id\": 0,\n        \"name\": \"Mckay Skinner\"\n      },\n      {\n        \"id\": 1,\n        \"name\": \"Amalia Valdez\"\n      },\n      {\n        \"id\": 2,\n        \"name\": \"Vazquez Cox\"\n      }\n    ],\n    \"greeting\": \"Hello, Little Beck! You have 3 unread messages.\",\n    \"favoriteFruit\": \"banana\"\n  },\n  {\n    \"_id\": \"59b53bcbd3aa145075803296\",\n    \"index\": 52,\n    \"guid\": \"bb4f7000-690a-4c88-be2f-37aaf08d774a\",\n    \"isActive\": false,\n    \"balance\": \"$3,595.09\",\n    \"picture\": \"http://placehold.it/32x32\",\n    \"age\": 37,\n    \"eyeColor\": \"green\",\n    \"name\": \"Alexander Jensen\",\n    \"gender\": \"male\",\n    \"company\": \"QUILK\",\n    \"email\": \"alexanderjensen@quilk.com\",\n    \"phone\": \"+1 (939) 458-3826\",\n    \"address\": \"911 Mill Street, Wyoming, Palau, 9790\",\n    \"about\": \"Ex nostrud id qui pariatur ex dolor velit adipisicing consectetur sit velit ullamco do. Reprehenderit incididunt labore commodo Lorem ex. Ea excepteur ullamco velit id non. Aliquip exercitation pariatur ullamco fugiat ad ipsum aute. Ipsum reprehenderit et consectetur eiusmod reprehenderit id. Aute eiusmod eu id do ut incididunt dolor occaecat cupidatat labore excepteur enim commodo deserunt.\\r\\n\",\n    \"registered\": \"2014-08-29T01:54:27 -01:00\",\n    \"latitude\": -67.074581,\n    \"longitude\": 64.927721,\n    \"tags\": [\n      \"cupidatat\",\n      \"nisi\",\n      \"tempor\",\n      \"reprehenderit\",\n      \"id\",\n      \"eiusmod\",\n      
